vi "xbox_360_joystick.vi"() -> ()   [LabVIEW 2016]
uses:
  <vilib>/Utility/inputDevices.llb/joystickAcquire.vi
  <vilib>/Utility/inputDevices.llb/closeJoystick.vi
panel:
  out "z axis info":i32
  out "y axis info":i32
  out "Y pressed":bool
  out "X pressed":bool
  out "B pressed":bool
  out "error out":errorcluster
  out "A pressed":bool
  out "dir info":i32
  out "x axis info":i32
  in  "Stop":bool
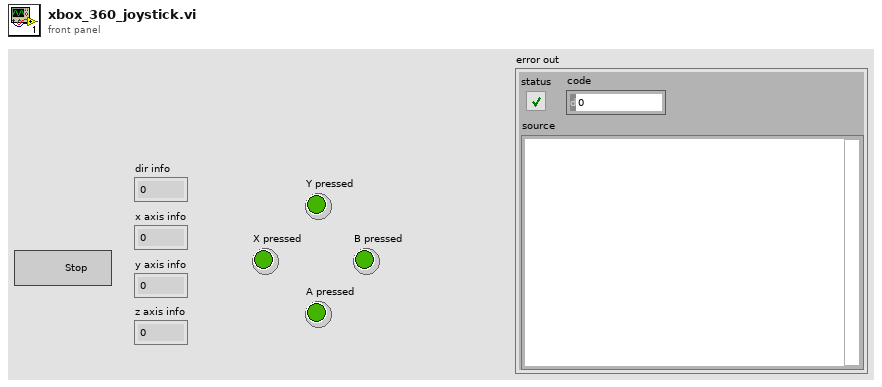
[diagram p1: front panel]
types:
  T1 = cluster{"X axis":i32, "Y axis":i32, "Z axis":i32, "X axis rotation":i32, "Y axis rotation":i32, "Z axis rotation":i32, "U axis":i32, "V axis":i32}
  T2 = cluster{"button 1":bool, "button 2":bool, "button 3":bool, "button 4":bool, "button 5":bool, "button 6":bool, "button 7":bool, "button 8":bool, "button 9":bool, "button 10":bool, "button 11":bool, "button 12":bool, "button 13":bool, "button 14":bool, "button 15":bool, "button 16":bool, "button 17":bool, "button 18":bool, "button 19":bool, "button 20":bool, "button 21":bool, "button 22":bool, "button 23":bool, "button 24":bool, "button 25":bool, "button 26":bool, "button 27":bool, "button 28":bool, "button 29":bool, "button 30":bool, "button 31":bool, "button 32":bool}
  T3 = cluster{"pov 1":i32, "pov 2":i32, "pov 3":i32, "pov 4":i32}
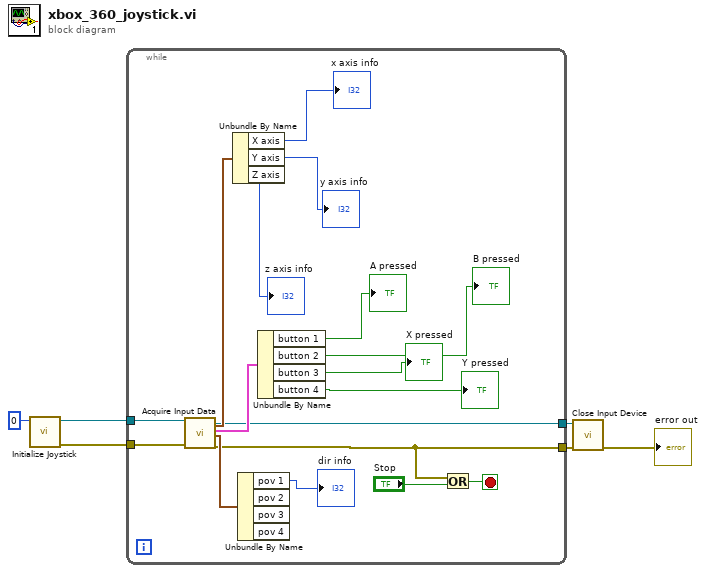
[diagram p0: block diagram]
diagram:
  n1 = call <vilib>:"Initialize Joystick.vi"("device index"=0) -> ("error out"=w5:errorcluster, "device ID"=w6:refnum<k1>)  [unwired: 9 in]
  n2 = while {
    tunnel: w6 -> [w23]
    tunnel: w5 -> [w16]
    tunnel: [w13] -> w3
    tunnel: [w12] -> w1
    stop <- w15 stop-if-true
    n3 = call-poly <vilib>:"Acquire Input Data.vi"("device ID"=w23, "error in (no error)"=w16) -> ("device ID"=w12:refnum<k1>, "axis info"=w22:T1, "button info"=w21:T2, "direction info"=w20:T3, "error out"=w13:errorcluster)  [unwired: 13 in]
    n4 = Unbundle By Name(w22) -> ("X axis"=→"x axis info":i32, "Y axis"=→"y axis info":i32, "Z axis"=→"z axis info":i32)
    n5 = Unbundle By Name(w20) -> ("pov 1"=→"dir info":i32)  [unwired: 3 out]
    n6 = Unbundle By Name(w21) -> ("button 1"=→"A pressed":bool, "button 2"=→"B pressed":bool, "button 3"=→"X pressed":bool, "button 4"=→"Y pressed":bool)
    n7 = Or(x=w13, y="Stop") -> (x .or. y?=w15:bool)
  }
  n8 = call-poly <vilib>:"Close Input Device.vi"("error in (no error)"=w3, "device ID"=w1) -> ("error out"=→"error out":errorcluster)  [unwired: 8 in]
